vi "Mix Secret Number.vi"(10 "Value":u64, 11 "Current Secret Number":u64) -> (3 "New Secret Number":u64)   [LabVIEW 2024]
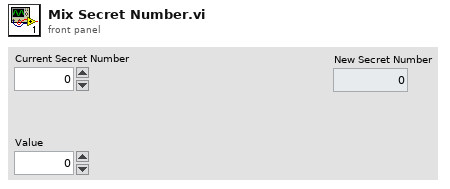
[diagram p1: front panel]
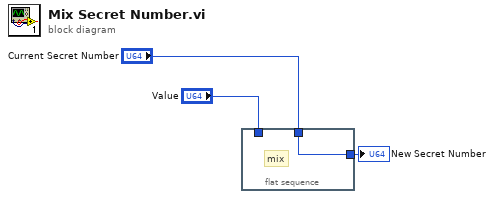
[diagram p0: block diagram]
diagram:
  n1 = flat-sequence {
    tunnel: "Value" -> [_]
    tunnel: "Current Secret Number" -> [w4]
    tunnel: [w4] -> w3
    frame #0 {
      # "mix"
    }
  }
  "New Secret Number" <- w3
